vi "Check Dispenser Communication.vi"   [LabVIEW 2016]
uses:
  Drivers/EFD Ultimus V/EFD Ultimus V.lvlib
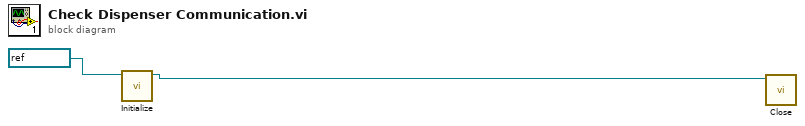
[diagram p0: block diagram]
diagram:
  n1 = call "Initialize.vi"("VISA resource name"=refnum<visa-resource-name> "COM1") -> ("VISA resource name out"=w1:refnum<visa-resource-name>)  [unwired: 9 in, 1 out]
  n2 = call "Close.vi"("VISA resource name"=w1) -> ()  [unwired: 10 in, 1 out]
